vi "Create Tolerance Bands.vi"(0 "DesiredCluster":T1, 7 "Tolerances":dbl[](array[numeric])) -> (4 "BoundsArray":dbl[][](array[numeric]))   [LabVIEW 2013]
uses:
  TypeDef/Command Cluster.ctl
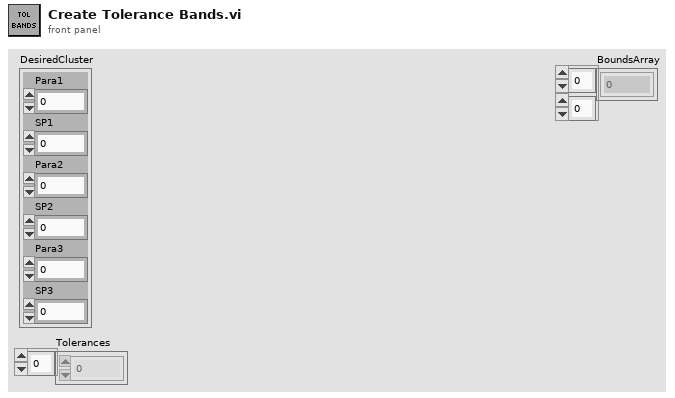
[diagram p1: front panel]
types:
  T1 = typedef "Command Cluster.ctl" = cluster{"Para1":i32, "SP1":dbl, "Para2":i32, "SP2":dbl, "Para3":i32, "SP3":dbl}
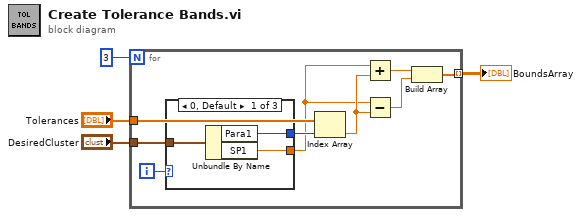
[diagram p0: block diagram]
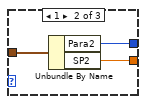
[diagram p2: hidden frame]
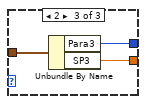
[diagram p3: hidden frame]
diagram:
  n1 = for {
    N: 3 -> [_]
    tunnel: "DesiredCluster" -> [w12]
    tunnel: "Tolerances" -> [w7]
    tunnel: [w8] -> w2 mode=indexing
    i -> [w13]
    n2 = case shown="0, Default" w13 {
      tunnel: w12 -> [w16 w19 w22]
      tunnel: [w15 w17 w21] -> w6
      tunnel: [w14 w18 w20] -> w5
      frame 0, Default {
        n3 = Unbundle By Name(w16) -> ("Para1"=w15:i32, "SP1"=w14:dbl)
      }
      frame 1 {
        n4 = Unbundle By Name(w19) -> ("Para2"=w17:i32, "SP2"=w18:dbl)
      }
      frame 2 {
        n5 = Unbundle By Name(w22) -> ("Para3"=w21:i32, "SP3"=w20:dbl)
      }
    }
    n6 = Index Array(array=w7, index=w6) -> (element=w9:dbl)
    n7 = Add(x=w5, y=w9) -> (x+y=w10:dbl)
    n8 = Subtract(x=w5, y=w9) -> (x-y=w11:dbl)
    n9 = Build Array(w10, w11) -> (w8:dbl[])
  }
  "BoundsArray" <- w2
